vi "Freefield-Initialize Measurement (TDT).vi"(0 "Endpoint":T1, 5 "Mic":string, 7 "Stimulus":T2, 11 "error in (no error)":errorcluster) -> (3 "Stimulus":dbl[](array[numeric]), 4 "RPcoX out":refnum<k7>, 12 "df (Hz)":dbl, 13 "dt (ms)":dbl, 14 "Mic Avg":dbl[](array[numeric]), 15 "error out":errorcluster)   [LabVIEW 2020]
uses:
  Common VIs/Typedefs/CAL-Stimulus.ctl
  Common VIs/Typedefs/CAL-Endpoint.ctl
  epl-vi-lib/PXI DAQ VIs/TDT VIs/TDT-Signal Bank Action.ctl
  2b0b6311-1651-4dbd-8b9d-77574cb074c4.vi
  5c07491a-2ef0-4b2f-b985-34a9a43085c4.vi
  <vilib>/Comparison/Equal/Equal Functor/Equal Functor.lvclass
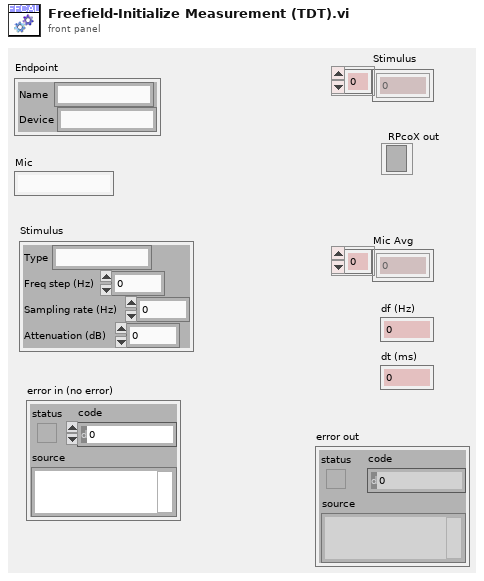
[diagram p1: front panel]
types:
  T1 = typedef "CAL-Endpoint.ctl" = cluster{"Name":string, "Device":string}
  T2 = typedef "CAL-Stimulus.ctl" = cluster{"Type":string, "Freq step (Hz)":dbl, "Sampling rate (Hz)":dbl, "Attenuation (dB)":dbl}
  T3 = typedef "TDT-Signal Bank Action.ctl" = enum16{"Init", "Write", "Read", "Rewrite", "Reset", "Recycle", "Ramp up", "Ramp down", "Zero"}
  T4 = typedef "TDT-Output source.ctl" = cluster{"Device":T5, "Num":i32}
  T5 = typedef "TDT-Device ID.ctl" = enum16{"None", "PA5", "RP2", "RL2", "RA16", "RV8", "RX5", "RX6", "RX7", "RX8", "RZ2", "RZ5", "RZ6"}
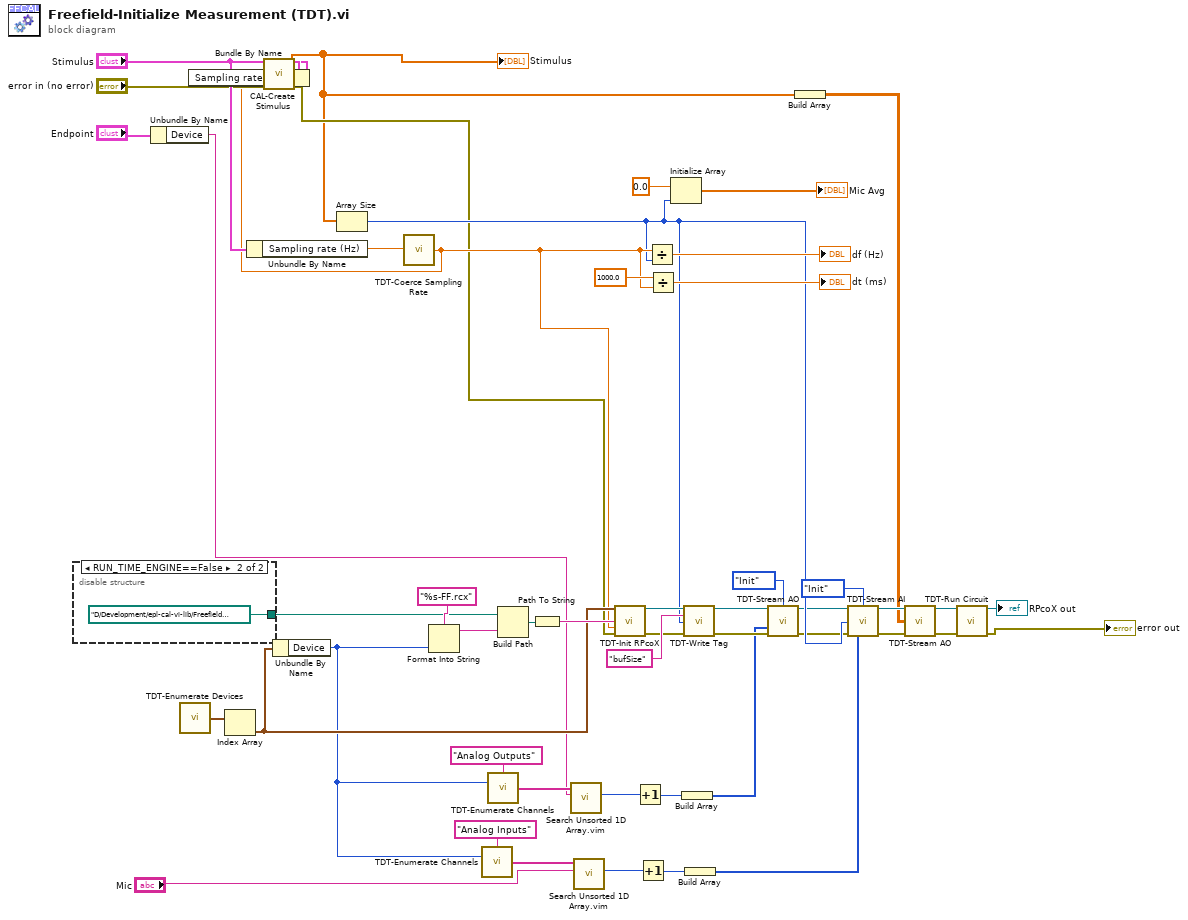
[diagram p0: block diagram]
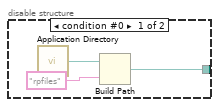
[diagram p2: hidden frame]
diagram:
  n1 = disable-structure shown="RUN_TIME_ENGINE==False" {
    disable-tunnel: [w52 path "D:/Development/epl-cal-vi-lib/Freefield Calibration VIs/rpfiles"] -> w38
    frame condition #0 {
      n2 = call <vilib>:"Application Directory.vi"() -> ("Application Directory"=w53:path)
      n3 = Build Path(base path=w53, name or relative path="rpfiles") -> (appended path=w52:path)
    }
    frame condition #1 (active) {
    }
  }
  n4 = Unbundle By Name("Endpoint") -> ("Device"=w4:string)
  n5 = call "TDT-Enumerate Devices.vi"() -> ("Devices"=w39:T4[])  [unwired: 14 in, 1 out]
  n6 = Index Array(array=w39) -> (element=w36:T4)  [unwired: 1 in]
  n7 = Unbundle By Name("Stimulus") -> ("Sampling rate (Hz)"=w25:dbl)
  n8 = Unbundle By Name(w36) -> ("Device"=w8:T5)
  n9 = call "TDT-Coerce Sampling Rate.vi"("Fs (Hz)"=w25) -> ("Coerced"=w23:dbl)
  n10 = Bundle By Name(cluster="Stimulus", "Sampling rate (Hz)"=w23) -> (w24:T2)
  n11 = call "CAL-Create Stimulus.vi"("Cal Stimulus"=w24, "error in (no error)"="error in (no error)") -> ("Stimulus"=w2:dbl[], "error out"=w11:errorcluster)  [unwired: 12 in]
  "Stimulus" <- w2
  n12 = Array Size(array=w2) -> (size(s)=w22:i32)
  n13 = Format Into String(format string="%s-FF.rcx", w8) -> (resulting string=w41:string)  [unwired: 2 in, 1 out]
  n14 = call "TDT-Enumerate Channels.vi"("Type"="Analog Inputs", "IO Device"=w8) -> ("IO Channels"=w31:string[])  [unwired: 13 in]
  n15 = call "TDT-Enumerate Channels.vi"("Type"="Analog Outputs", "IO Device"=w8) -> ("IO Channels"=w5:string[])  [unwired: 13 in]
  n16 = Build Path(base path=w38, name or relative path=w41) -> (appended path=w40:path)
  n17 = Path To String(path=w40) -> (string=w37:string)
  n18 = call "Search Unsorted 1D Array.vim"("element"=w4, "unsorted 1D array"=w5) -> ("index of element"=w7:i32)  [unwired: 9 in]
  n19 = call "Search Unsorted 1D Array.vim"("element"="Mic", "unsorted 1D array"=w31) -> ("index of element"=w29:i32)  [unwired: 9 in]
  n20 = call "TDT-Init RPcoX.vi"("Output"=w36, "RPfilename"=w37, "Sampling rate (Hz)"=w23, "error in (no error)"=w11) -> ("RPcoX"=w35:refnum<k7>, "error out"=w33:errorcluster)  [unwired: 10 in]
  n21 = Increment(x=w7) -> (x+1=w6:i32)
  n22 = Increment(x=w29) -> (x+1=w28:i32)
  n23 = Divide(x=w23, y=w22) -> (x/y=→"df (Hz)":dbl)
  n24 = Divide(x=1000.0, y=w23) -> (x/y=→"dt (ms)":dbl)
  n25 = Initialize Array(0.0 ("element"), w22) -> (→"Mic Avg":dbl[])
  n26 = Build Array(w6) -> (w3:i32[])
  n27 = call "TDT-Write Tag.vi"("RPcox"=w35, "Name"="bufSize", "Value"=w22, "error in"=w33) -> ("RPcox Out"=w20:refnum<k7>, "error out"=w18:errorcluster)  [unwired: 10 in]
  n28 = Build Array(w28) -> (w27:i32[])
  n29 = call "TDT-Stream AO.vi"("RPcox"=w20, "Action"=TDT-Signal_Bank_Action."Init", "Chans"=w3, "error in (no error)"=w18) -> ("RPcox thru"=w19:refnum<k7>, "error out"=w17:errorcluster)  [unwired: 10 in]
  n30 = Build Array(w2) -> (w1:dbl[][])
  n31 = call "TDT-Stream AI.vi"("RPcox"=w19, "Action"=TDT-Signal_Bank_Action."Init", "Pts Per Read"=w22, "error in (no error)"=w17, "AI Channels"=w27) -> ("RPcoX thru"=w16:refnum<k7>, "error out"=w13:errorcluster)  [unwired: 8 in, 1 out]
  n32 = call "TDT-Stream AO.vi"("RPcox"=w16, "Output array"=w1, "error in (no error)"=w13) -> ("RPcox thru"=w15:refnum<k7>, "error out"=w14:errorcluster)  [unwired: 11 in]
  n33 = call "TDT-Run Circuit.vi"("RPcoX"=w15, "error in (no error)"=w14) -> ("RPcoX out"=→"RPcoX out":refnum<k7>, "error out"=→"error out":errorcluster)  [unwired: 12 in]
